vi "电脑关机.vi"   [LabVIEW 2016]
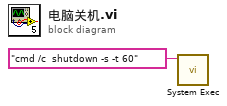
[diagram p0: block diagram]
diagram:
  n1 = call <vilib>:"System Exec.vi"("command line"="cmd /c  shutdown -s -t 60") -> ()  [unwired: 7 in, 4 out]
